vi "000 Write Convert.vi"(10 "Name In":string, 11 "Formular":string) -> (2 "Name Out":string)   [LabVIEW 2020]
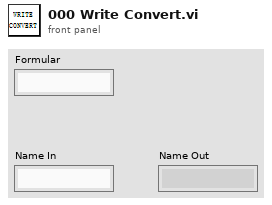
[diagram p1: front panel]
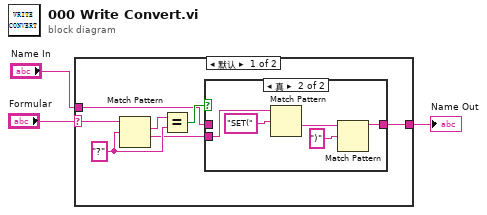
[diagram p0: block diagram]
diagram:
  n1 = case shown="默认" "Formular" {
    selector: "Formular" -> [w10 _]
    tunnel: "Name In" -> [w5 w17]
    tunnel: [w4 w17] -> w1
    frame Default {
      w8 = "?" ("正则表达式")
      n2 = Match Pattern(string=w10, regular expression=w8) -> (match substring=w9:string, after substring=w6:string)  [unwired: 1 in, 2 out]
      n3 = Equal?(x=w9, y=w8) -> (x = y?=w7:bool)
      n4 = case shown="真" w7 {
        tunnel: w6 -> [_ w16]
        tunnel: [w11 w12] -> w4
        tunnel: w5 -> [w11 _]
        frame False {
        }
        frame True {
          n5 = Match Pattern(string=w16, regular expression="SET(" ("正则表达式")) -> (after substring=w14:string)  [unwired: 1 in, 3 out]
          n6 = Match Pattern(string=w14, regular expression=")" ("正则表达式")) -> (before substring=w12:string)  [unwired: 1 in, 3 out]
        }
      }
    }
    frame "" {
    }
  }
  "Name Out" <- w1
